vi "write memory.vi"(8 "error in (no error)":errorcluster, 10 "IQ data":u64[](array[numeric]), 11 "5785_2_x_1600MHz in":refnum<class "5785_2_x_1600MHz.lvclass">) -> (0 "error out":errorcluster, 3 "5785_2_x_1600MHz out":refnum<class "5785_2_x_1600MHz.lvclass">)   [LabVIEW 2021, in "5785_2_x_1600MHz.lvclass"]
uses:
  5785_2_x_1600MHz.lvclass
  5785_2_x_1600MHz.lvclass/5785_2_x_1600MHz.ctl
  <vilib>/Utility/error.llb/Error Cluster From Error Code.vi
  <vilib>/rvi/errors/niLvFpgaAdjustHostInterfaceError.vi
  <vilib>/rvi/interface/nirviMethod/nirviMethod.xnode
  <vilib>/FPGAPlugInAG/Dynamic/niLvFpga_WriteFifo_Dynamic.vi
  <vilib>/rvi/errors/niLvFpgaMergeErrorWithErrorCode.vi
  <vilib>/FPGAPlugInAG/Dynamic/niLvFpga_ConfigureFifo_Dynamic.vi
  <vilib>/FPGAPlugInAG/Dynamic/niLvFpga_StopFifo_Dynamic.vi
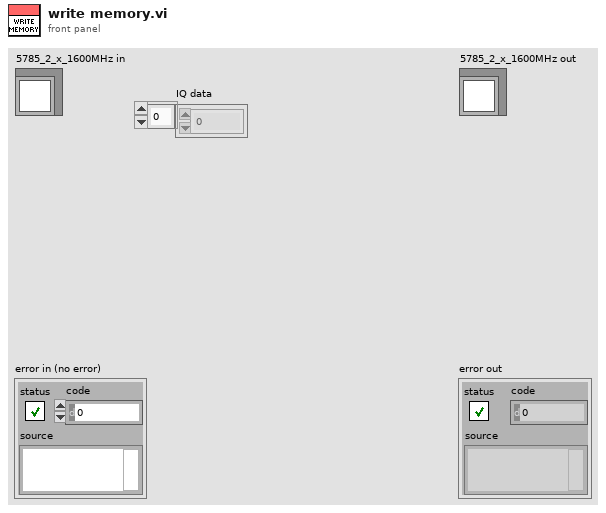
[diagram p1: front panel]
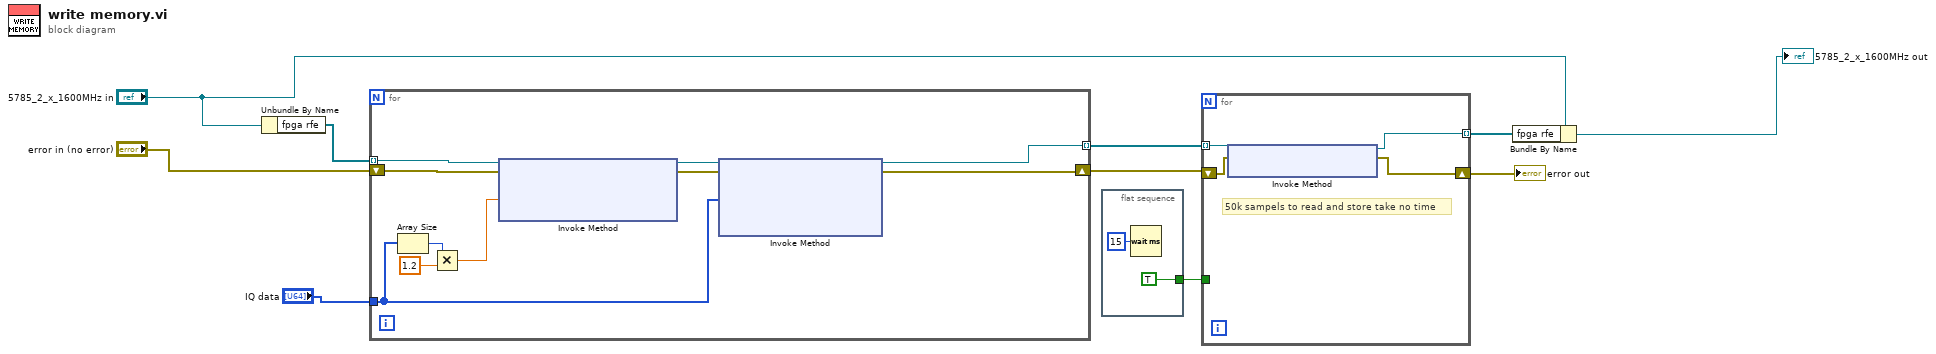
[diagram p0: block diagram]
diagram:
  n1 = Unbundle By Name("5785_2_x_1600MHz in") -> ("fpga rfe"=w10:refnum<k20>[])
  n2 = for {
    tunnel: w10 -> [w14] mode=indexing
    tunnel: "IQ data" -> [w18]
    shift-right: [w19] -> w2
    shift-left: "error in (no error)" -> [w13]
    tunnel: [w20] -> w5 mode=indexing
    n3 = Array Size(array=w18) -> (size(s)=w17:i32)
    n4 = Multiply(x=w17, y=1.2) -> (x*y=w16:dbl)
    n5 = xnode "Invoke Method"("FPGA VI Reference In"=w14, "error in"=w13, "Requested Depth"=w16) -> ("FPGA VI Reference Out"=w12:refnum<k20>, "error out"=w11:errorcluster)  [unwired: 1 out]
    n6 = xnode "Invoke Method"("FPGA VI Reference In"=w12, "error in"=w11, "Data"=w18) -> ("FPGA VI Reference Out"=w20:refnum<k20>, "error out"=w19:errorcluster)  [unwired: 1 in, 1 out]
  }
  n7 = flat-sequence {
    tunnel: [TRUE] -> w1
    frame #0 {
      n8 = Wait (ms)(milliseconds to wait=u32 15) -> ()  [unwired: 1 out]
    }
  }
  n9 = for {
    tunnel: w5 -> [w26] mode=indexing
    tunnel: [w24] -> w4 mode=indexing
    shift-right: [w23] -> w3
    shift-left: w2 -> [w25]
    tunnel: w1 -> [_]
    # "50k sampels to read and store take no time"
    n10 = xnode "Invoke Method"("FPGA VI Reference In"=w26, "error in"=w25) -> ("FPGA VI Reference Out"=w24:refnum<k20>, "error out"=w23:errorcluster)
  }
  "error out" <- w3
  n11 = Bundle By Name(cluster="5785_2_x_1600MHz in", "fpga rfe"=w4) -> (→"5785_2_x_1600MHz out":refnum<class "5785_2_x_1600MHz.lvclass">)
